vi "Update Status Message for Test.vi"(11 "MTS Radio Test in":refnum<class "MTS Radio Test.lvclass">) -> ()   [LabVIEW 2015, in "MTS Radio Test.lvclass"]
uses:
  MTS Radio Test.lvclass
  Test Class/Test Class.lvclass
  Classes/Application/Class/Application.lvclass
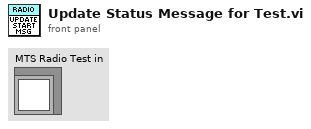
[diagram p1: front panel]
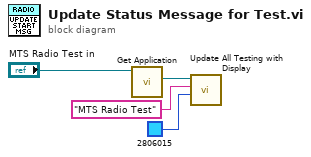
[diagram p0: block diagram]
diagram:
  n1 = call "Get Application.vi"("Test Class in"="MTS Radio Test in") -> ("Application.lvlib:Application.lvclass"=w4:refnum<class "Application.lvclass">)  [unwired: 9 in, 1 out]
  n2 = call "Update All Testing with Display.vi"("BG Color"=u32 2806015, "Message ('')"="MTS Radio Test", "Application in"=w4) -> ()  [unwired: 7 in, 2 out]
